vi "Send RFSG Trigger.vi"(8 "error in (no error)":errorcluster, 11 "rfsg queue":refnum<queue>) -> (0 "error out":errorcluster)   [LabVIEW 2021]
uses:
  Messaging/RFSG Message.ctl
  RFSG Configuration.ctl
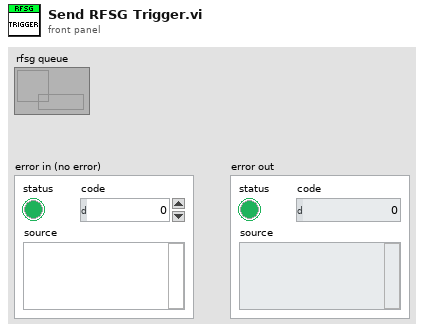
[diagram p1: front panel]
types:
  T1 = typedef "RFSG Message.ctl" = enum16{"Trigger Ready", "Run RF", "Stop RF", "Exit"}
  T2 = typedef "RFSG Configuration.ctl" = cluster{"rfsg ref":refnum<k15>, "freq off":i32, "wfm type":u16, "cent freq":dbl, "iq rate":dbl, "power":dbl, "msg":T1}
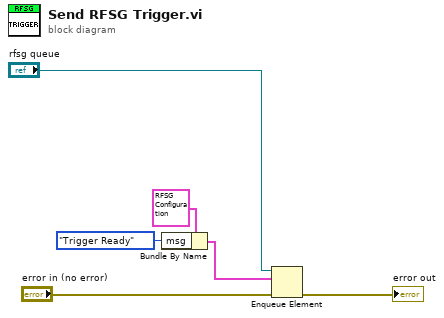
[diagram p0: block diagram]
diagram:
  n1 = Bundle By Name(cluster=T2 {"rfsg ref"="5646VST", "freq off"=2, "wfm type"=0, "cent freq"=1000000000.0, "iq rate"=2000000.0, "power"=-10.0, "msg"=enum."Trigger Ready"} ("element"), "msg"=RFSG_Message."Trigger Ready") -> (w1:T2)
  n2 = Enqueue Element(queue="rfsg queue", element=w1, error in (no error)="error in (no error)") -> (error out=→"error out":errorcluster)  [unwired: 1 in, 2 out]
